vi "SRV_In PicoC State Change.vi"(9 "In Pico":bool, 10 "InPico State Change":bool) -> (1 "Read PicoC Buffer?":bool, 2 "InPico State Change out":bool)   [LabVIEW 2014]
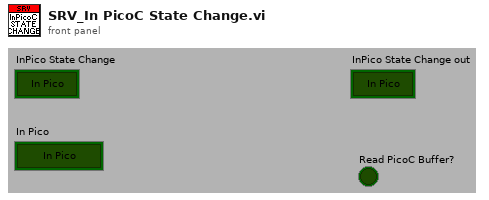
[diagram p1: front panel]
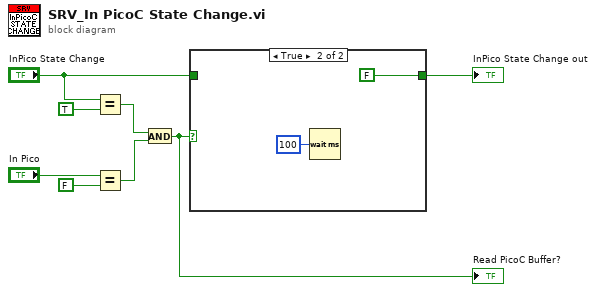
[diagram p0: block diagram]
diagram:
  n1 = Equal?(x="InPico State Change", y=TRUE) -> (x = y?=w5:bool)
  n2 = Equal?(x="In Pico", y=FALSE) -> (x = y?=w4:bool)
  n3 = And(x=w5, y=w4) -> (x .and. y?=w1:bool)
  "Read PicoC Buffer?" <- w1
  n4 = case shown="True" w1 {
    tunnel: "InPico State Change" -> [w9 _]
    tunnel: [w9 FALSE ("InPico State Change")] -> w2
    frame False {
    }
    frame True {
      n5 = Wait (ms)(milliseconds to wait=u32 100) -> ()  [unwired: 1 out]
    }
  }
  "InPico State Change out" <- w2
